vi "data-center-monitor.vi"() -> ()   [LabVIEW 2024]
doc: "Demonstrates how to implement advanced power measurement of harmonic parameters on a three-phase electrical power system, such as measurement of harmonic distortion factor, total harmonic distortion, harmonic power, etc. Measurement of harmonic parameters is based on a resampling algorithm."
uses:
  <vilib>/addons/Electrical Power/Power Measurement/subVIs/ep_Resampled Data.ctl
  <vilib>/Utility/error.llb/DialogType.ctl
  <vilib>/DAQmx/read.llb/DAQmx Read (Analog 1D Wfm NChan NSamp).vi
  <extravilib>/ChannelInstances/Tag-bool/Read.vi
  <extravilib>/ChannelInstances/Tag-bool/Write.vi
  <extravilib>/ChannelInstances/Tag-bool/Read With Abort.vi
  <extravilib>/ChannelInstances/Tag-bool/Write With Abort.vi
  <vilib>/DAQmx/create/channels.llb/DAQmx Create Channel (AI-Voltage-Basic).vi
  <vilib>/DAQmx/create/channels.llb/DAQmx Create Channel (AI-Current-Basic).vi
  <vilib>/DAQmx/configure/timing.llb/DAQmx Timing (Sample Clock).vi
  <extravilib>/ChannelInstances/Tag-bool/Instantiate.vi
  <vilib>/addons/Electrical Power/Basic/Measurement/Fundamental Vector (N Channels).vi
  <extravilib>/ChannelInstances/Tag-bool/EndpointRead.vi
  <extravilib>/ChannelInstances/Tag-bool/Endpoint.vi
  <vilib>/DAQmx/miscellaneous.llb/DAQmx Fill In Error Info.vi
  <resource>/objmgr/daqmx.rc
  <vilib>/addons/Electrical Power/Power Measurement/NI_EP_Power Measurement.lvlib
  <vilib>/addons/Electrical Power/Basic/NI_EP_Basic.lvlib
panel:
  in  "Display":T1(tab)
  in  "Configuration":enum32{"DAQmx", "Others"}(tab)
  in  "number of samples per channel":i32=10000
  in  "DAQmx sample rate [Hz]":dbl=50000.0 format="%0.2f"
  in  "current channels":tag="current-input/ai0:2"
  in  "maximum current value":dbl=0.002 format="%0.3f"
  in  "minimum current value":dbl=-0.002 format="%0.3f"
  in  "voltage channels":tag="voltage-input/ai0:2"
  in  "maximum voltage value":dbl=300.0 format="%0.2f"
  in  "minimum voltage value":dbl=-300.0 format="%0.2f"
  in  "frequency range [Hz]":cluster{"minimum":dbl, "maximum":dbl}={"minimum"=45.0, "maximum"=65.0}
  in  "samples per cycle":u16=192
  in  "cycles per block":u16=10
  in  "maximum harmonic  order":u16=50
  in  "distortion factor denominator":enum16{"Fundamental value", "Total value"}(ring)
  in  "filter for frequency measurement":T2={"enable filter? (T)"=TRUE, "passband edge frequency [Hz]"=65.0, "passband ripple [dB]"=0.1, "stopband edge frequency [Hz]"=85.0, "stopband attenuation [dB]"=60.0}
  out "Service Rack":cluster{dbl[], dbl[]}[](graph)
  out "PDU":cluster{dbl[], dbl[]}[](graph)
  out "V THD [%]":dbl[](array[numeric]) format="%#_2g"
  out "I THD [%]":dbl[](array[numeric]) format="%#_2g"
  out "Average Frequency [Hz]":dbl format="%#_3g"
  out "Power Usage":T3(graph)
  out "actual DAQmx \nsample rate  [Hz]":dbl
  out "average frequency [Hz]":dbl
  out "Waveforms":T4(graph)
  out "Voltage Harmonic Spectra":T5(graph)
  out "Current Harmonic Spectra":T5(graph)
  out "voltage total values":dbl[](array[numeric])
  out "voltage THD [%]":dbl[](array[numeric])
  out "voltage harmonic distortion factors [%]":dbl[][](array[numeric])
  out "current THD [%]":dbl[](array[numeric])
  out "total power value":T6
  out "harmonic power values":T7(array[cluster])
  out "power values":T3(array[cluster])
  out "Fundamental Voltage Vectors (Vrms)":cluster{dbl[], dbl[]}[](graph)
  out "Fundamental Current Vectors (Arms)":cluster{dbl[], dbl[]}[](graph)
  out "power history":T3(graph)
  in  "pause-update":bool
  in  "stop":bool
  # "Data Center Power Monitor Demo"
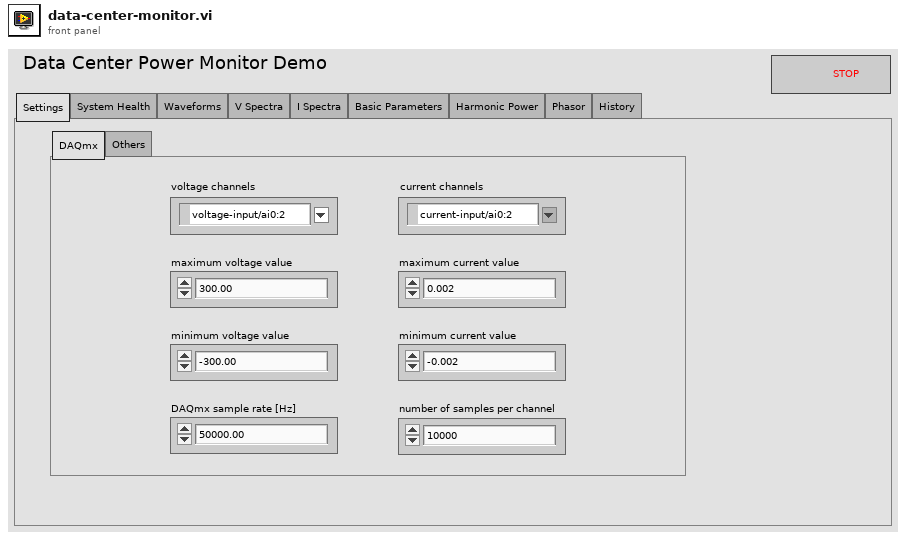
[diagram p1: front panel]
types:
  T1 = enum32{"Settings", "System Health", "Waveforms", "V Spectra", "I Spectra", "Basic Parameters", "Harmonic Power", "Phasor", "History"}
  T2 = cluster{"enable filter? (T)":bool, "passband edge frequency [Hz]":dbl, "passband ripple [dB]":dbl, "stopband edge frequency [Hz]":dbl, "stopband attenuation [dB]":dbl}
  T3 = cluster{"active power [W]":dbl, "apparent power [VA]":dbl, "reactive power [VAR]":dbl, "power factor":dbl}[]
  T4 = cluster{"positions [s]":dbl[], "resampled signal":dbl[]}[]
  T5 = cluster{"order 0":dbl, "delta order":dbl, "complex spectrum":dbl[]}[]
  T6 = cluster{"active power [W]":dbl, "apparent power [VA]":dbl, "reactive power [VAR]":dbl, "power factor":dbl}
  T7 = cluster{"active power [W]":dbl, "apparent power [VA]":dbl, "reactive power [VAR]":dbl, "power factor":dbl}[][]
  T8 = typedef "DialogType.ctl" = u16
  T9 = typedef "NI_EP_Power Measurement.lvlib/ep_Resampled Data.ctl" = cluster{"times [s]":dbl[], "resampled signal":dbl[]}
  T10 = cluster{"zero crossing times [s]":dbl[], "zero crossings per cycle":u8}
  T11 = typedef "Tag-bool.lvlib/))Channel.ctl" = refnum<queue>
  T12 = cluster{"order 0":dbl, "delta order":dbl, "complex spectrum":cdb[]}[]
  T13 = typedef "NI_EP_Basic.lvlib/basic_Power Value.ctl" = cluster{"active power [W]":dbl, "apparent power [VA]":dbl, "reactive power [VAR]":dbl, "power factor":dbl}
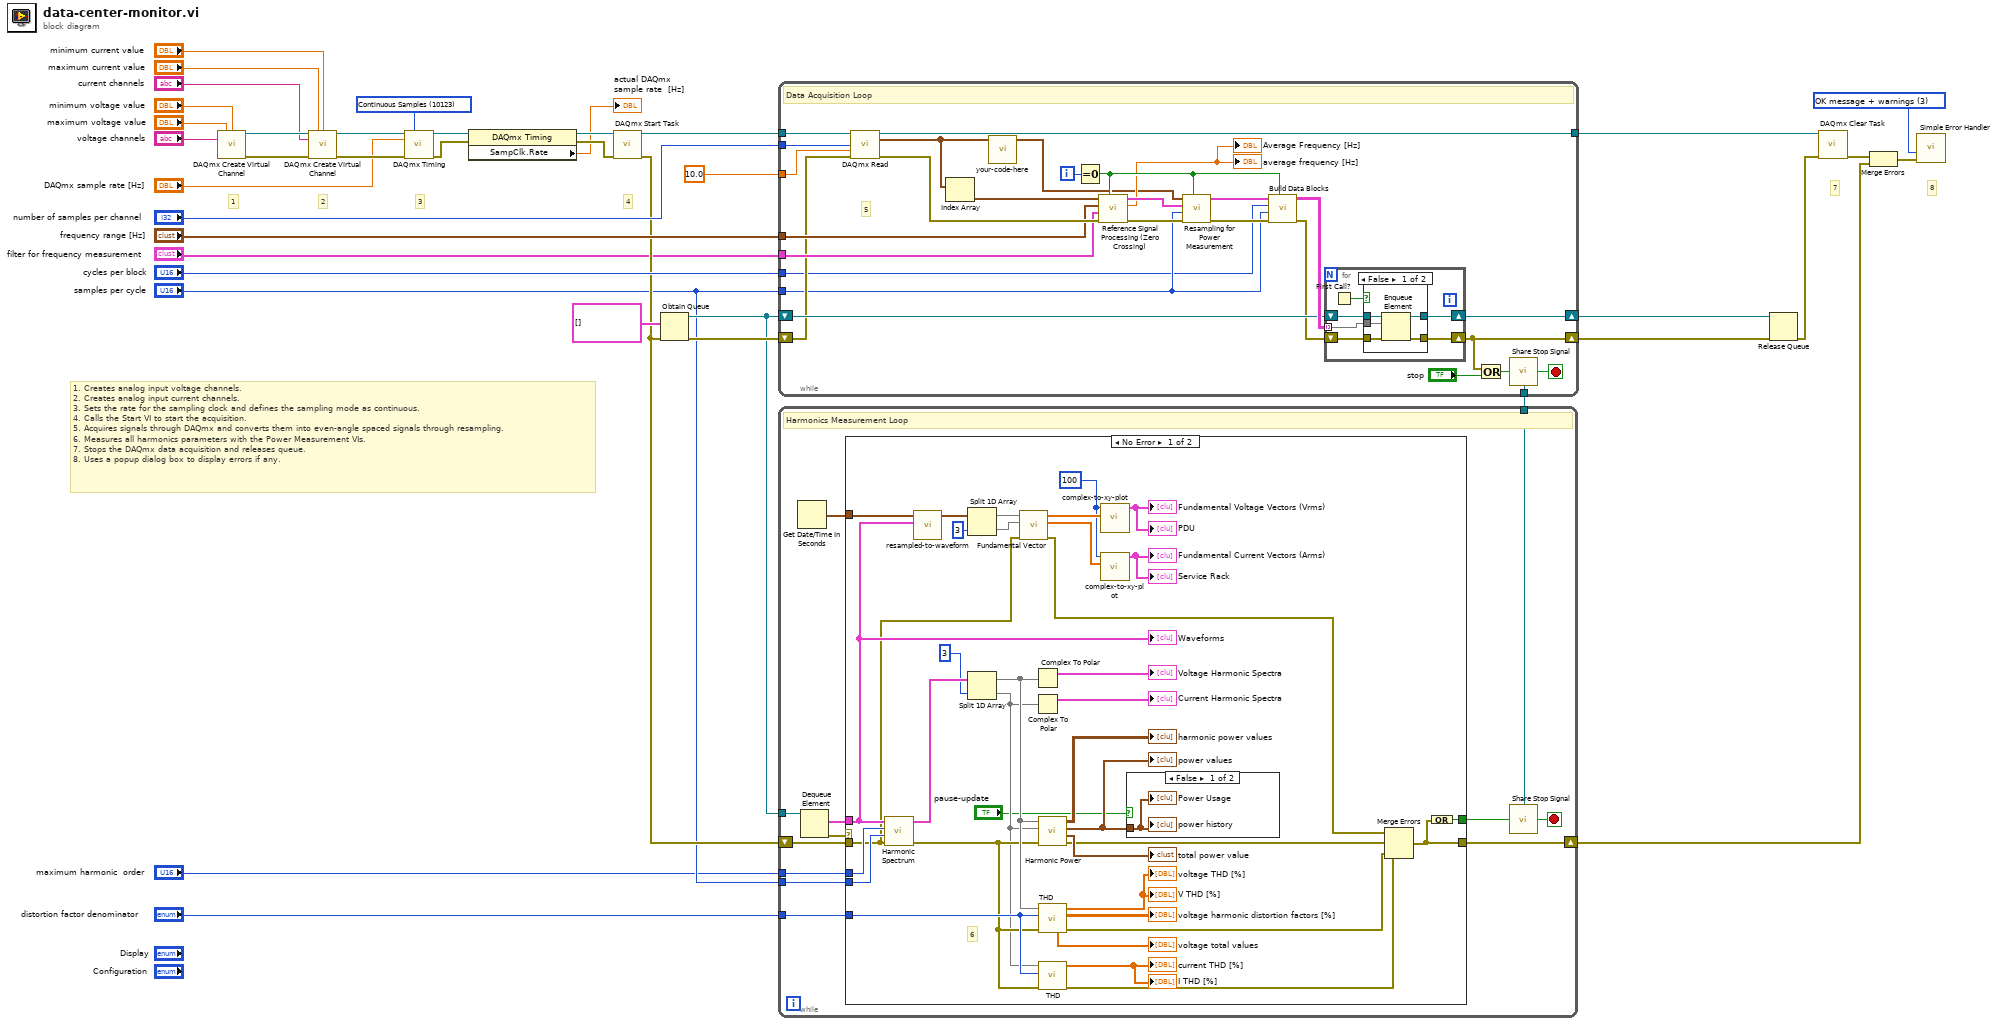
[diagram p0: block diagram]
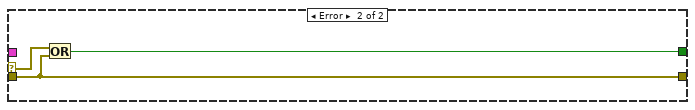
[diagram p3: hidden frame]
diagram:
  w6 = T8 3 items=["no dialog", "OK message", "continue or stop message", "OK message + warnings", "continue/stop + warnings"] ("type of dialog (OK msg:1)")
  w8 = 10123 items=["Finite Samples"=10178, "Continuous Samples"=10123, "Hardware Timed Single Point"=12522] ("sample mode")
  # "8"
  # "7"
  # "1. Creates analog input voltage channels.\n2. Creates analog input current channels.\n3. Sets the rate for the sampling clock and defines the sampling mode as continuous.\n4. Calls the Start VI to start the acquisition.\n5. Acquires signals through DAQmx and converts them into even-angle spaced signals through resampling. \n6. Measures all harmonics parameters with the Power Measurement VIs.\n7.\tStops the DAQmx data acquisition and releases queue.\n8. Uses a popup dialog box to display errors if any."
  # "4"
  # "3"
  # "2"
  # "1"
  n1 = call-poly <vilib>:"DAQmx Create Virtual Channel.vi"("maximum value"="maximum voltage value", "minimum value"="minimum voltage value", "physical channels"="voltage channels") -> ("task out"=w35:refnum<k21>, "error out"=w36:errorcluster)  [unwired: 11 in]
  n2 = call-poly <vilib>:"DAQmx Create Virtual Channel.vi"("task in"=w35, "maximum value"="maximum current value", "minimum value"="minimum current value", "physical channels"="current channels", "error in"=w36) -> ("task out"=w30:refnum<k21>, "error out"=w31:errorcluster)  [unwired: 9 in]
  n3 = call-poly <vilib>:"DAQmx Timing.vi"("task/channels in"=w30, "sample mode"=w8, "rate"="DAQmx sample rate [Hz]", "error in"=w31) -> ("task out"=w24:refnum<k21>, "error out"=w28:errorcluster)  [unwired: 10 in]
  n4 = property class="DAQmx Timing"(reference=w24, error in=w28) -> (reference out=w27:refnum<k21>, error out=w26:errorcluster, "SampClk.Rate"=→"actual DAQmx \nsample rate  [Hz]":dbl)
  n5 = call <vilib>:"DAQmx Start Task.vi"("task/channels in"=w27, "error in"=w26) -> ("task out"=w25:refnum<k21>, "error out"=w14:errorcluster)  [unwired: 12 in]
  n6 = Obtain Queue(element data type=T9[] [] ("resampled data"), error in (no error)=w14) -> (queue out=w15:refnum<queue>, error out=w19:errorcluster)  [unwired: 3 in, 1 out]
  n7 = while {
    tunnel: "number of samples per channel" -> [w67]
    tunnel: w25 -> [w68]
    tunnel: [w66] -> w21
    tunnel: "frequency range [Hz]" -> [w62]
    tunnel: "filter for frequency measurement" -> [w61]
    shift-right: [w52] -> w17
    shift-left: w15 -> [w54]
    shift-right: [w44] -> w4
    shift-left: w19 -> [w53]
    tunnel: "samples per cycle" -> [w51]
    tunnel: "cycles per block" -> [w50]
    tunnel: 10.0 ("timeout") -> [w46]
    tunnel: [w40] -> w1
    i -> [w64]
    stop <- w47 stop-if-true
    # "5"
    # "Data Acquisition Loop"
    n8 = call-poly <vilib>:"DAQmx Read.vi"("task/channels in"=w68, "number of samples per channel"=w67, "timeout"=w46, "error in"=w53) -> ("task out"=w66:refnum<k21>, "data"=w42:waveform(dbl)[], "error out"=w65:errorcluster)  [unwired: 9 in]
    n9 = Index Array(array=w42) -> (element=w63:waveform(dbl))  [unwired: 1 in]
    n10 = call "your-code-here.vi"("data in"=w42) -> ("data out"=w41:waveform(dbl)[])  [unwired: 10 in]
    n11 = Equal To 0?(x=w64) -> (x = 0?=w56:bool)
    n12 = call <vilib>:"Reference Signal Processing (Zero Crossing).vi"("reset? (F)"=w56, "error in (no error)"=w65, "filter for frequency measurement"=w61, "frequency range [Hz]"=w62, "reference signal"=w63) -> ("error out"=w60:errorcluster, "average frequency [Hz]"=→"average frequency [Hz]" →"Average Frequency [Hz]":dbl, "zero crossing information"=w59:T10)  [unwired: 3 in, 1 out]
    n13 = call <vilib>:"Resampling for Power Measurement.vi"("reset? (F)"=w56, "error in (no error)"=w60, "samples per cycle (192)"=w51, "trigger information"=w59, "data in"=w41) -> ("error out"=w58:errorcluster, "resampled data"=w57:T9[])  [unwired: 5 in]
    n14 = call <vilib>:"Build Data Blocks.vi"("reset? (F)"=w56, "error in (no error)"=w58, "samples per cycle (192)"=w51, "cycles per block (10)"=w50, "resampled data"=w57) -> ("error out"=w45:errorcluster, "data blocks"=w55:T9[][])  [unwired: 5 in]
    n15 = for {
      shift-right: [w72] -> w52
      shift-left: w54 -> [w73]
      shift-right: [w74] -> w44
      shift-left: w45 -> [w71]
      tunnel: w55 -> [w70] mode=indexing
      n16 = First Call?() -> (First Call?: T/F=w69:bool)
      n17 = case shown="False" w69 {
        tunnel: [w79 w80] -> w74
        tunnel: w73 -> [w78 w81]
        tunnel: [w77 w81] -> w72
        tunnel: w71 -> [w76 w80]
        tunnel: w70 -> [w75 _]
        frame False {
          n18 = Enqueue Element(queue=w78, element=w75, error in (no error)=w76) -> (queue out=w77:refnum<queue>, error out=w79:errorcluster)  [unwired: 1 in, 1 out]
        }
        frame True {
        }
      }
    }
    n19 = Or(x=w44, y="stop") -> (x .or. y?=w48:bool)
    n20 = call <vilib>:"Share Stop Signal.vi"("set stop (F)"=w48) -> ("channel"=w40:T11, "stop"=w47:bool)
  }
  n21 = while {
    shift-right: [w85] -> w10
    shift-left: w14 -> [w88]
    tunnel: w15 -> [w93]
    tunnel: "samples per cycle" -> [w91]
    tunnel: "maximum harmonic  order" -> [w90]
    tunnel: "distortion factor denominator" -> [w89]
    tunnel: w1 -> [w82]
    stop <- w86 stop-if-true
    # "Harmonics Measurement Loop"
    n22 = Get Date/Time In Seconds() -> (seconds since 1Jan1904=w83:timestamp)
    n23 = Dequeue Element(queue=w93) -> (element=w92:T9[], error out=w87:errorcluster)  [unwired: 2 in, 2 out]
    n24 = case shown="No Error" w87 {
      selector: w87 -> [_ w133]
      tunnel: w92 -> [w112 _]
      tunnel: w91 -> [w129 _]
      tunnel: w90 -> [w128 _]
      tunnel: w88 -> [w103 w132]
      tunnel: [w120 w132] -> w85
      tunnel: w89 -> [w125 _]
      tunnel: [w114 w131] -> w84
      tunnel: w83 -> [w111 _]
      frame No Error {
        w104 = 100
        # "6"
        n25 = call <vilib>:"Harmonic Spectrum.vi"("error in (no error)"=w103, "samples per cycle (192)"=w129, "maximum harmonic order (50)"=w128, "resampled data"=w112) -> ("error out"=w115:errorcluster, "harmonic spectra"=w127:T12)  [unwired: 6 in]
        n26 = call "resampled-to-waveform.vi"("resampled data"=w112, "current-timestamp"=w111) -> ("waveform data"=w109:waveform(dbl)[])  [unwired: 9 in]
        n27 = Split 1D Array(array=w109, index=3) -> (first subarray=w108:waveform(dbl)[], second subarray=w107:waveform(dbl)[])
        n28 = Split 1D Array(array=w127, index=3) -> (first subarray=w126:T12, second subarray=w100:T12)
        n29 = call-poly <vilib>:"Fundamental Vector.vi"("error in (no error)"=w103, "current waveforms"=w107, "voltage waveforms"=w108) -> ("error out"=w102:errorcluster, "current fundamental vectors"=w105:cdb[], "voltage fundamental vectors"=w106:cdb[])  [unwired: 5 in, 1 out]
        n30 = Complex To Polar(r * e^(i*theta)=w126) -> (r=→"Voltage Harmonic Spectra":T5)  [unwired: 1 out]
        n31 = Complex To Polar(r * e^(i*theta)=w100) -> (r=→"Current Harmonic Spectra":T5)  [unwired: 1 out]
        n32 = call <vilib>:"Harmonic Power.vi"("error in (no error)"=w115, "current spectra"=w100, "voltage spectra"=w126) -> ("error out"=w121:errorcluster, "total power value"=→"total power value":T13, "power values"=w101:T13[], "harmonic power values"=→"harmonic power values":T13[][])  [unwired: 5 in]
        "power values" <- w101
        n33 = call <vilib>:"THD.vi"("error in (no error)"=w115, "distortion factor denominator"=w125, "harmonic spectra"=w126) -> ("error out"=w116:errorcluster, "harmonic distortion factors [%]"=→"voltage harmonic distortion factors [%]":dbl[][], "THD [%]"=→"voltage THD [%]" →"V THD [%]":dbl[], "total values"=→"voltage total values":dbl[])  [unwired: 5 in]
        n34 = call <vilib>:"THD.vi"("error in (no error)"=w115, "distortion factor denominator"=w125, "harmonic spectra"=w100) -> ("error out"=w119:errorcluster, "THD [%]"=→"current THD [%]" →"I THD [%]":dbl[])  [unwired: 5 in, 2 out]
        n35 = call "complex-to-xy-plot.vi"("complex-vector"=w106, "number-of-points"=w104) -> ("xy-plot-output"=→"Fundamental Voltage Vectors (Vrms)" →"PDU":cluster{dbl[], dbl[]}[])  [unwired: 9 in]
        n36 = call "complex-to-xy-plot.vi"("complex-vector"=w105, "number-of-points"=w104) -> ("xy-plot-output"=→"Fundamental Current Vectors (Arms)" →"Service Rack":cluster{dbl[], dbl[]}[])  [unwired: 9 in]
        n37 = case shown="False" "pause-update" {
          tunnel: w101 -> [w130 _]
          frame False {
            "power history" <- w130
            "Power Usage" <- w130
          }
          frame True {
          }
        }
        n38 = Merge Errors(w102, w121, w116, w119) -> (w120:errorcluster)
        n39 = Compound Arithmetic op=OR(w120) -> (w114:bool)
        "Waveforms" <- w112
      }
      frame Error {
        n40 = Or(x=w133, y=w132) -> (x .or. y?=w131:bool)
      }
    }
    n41 = call <vilib>:"Share Stop Signal.vi"("set stop (F)"=w84, "channel"=w82) -> ("stop"=w86:bool)
  }
  n42 = Release Queue(queue=w17, error in (no error)=w4) -> (error out=w3:errorcluster)  [unwired: 1 in, 2 out]
  n43 = call <vilib>:"DAQmx Clear Task.vi"("task in"=w21, "error in"=w3) -> ("error out"=w2:errorcluster)  [unwired: 13 in]
  n44 = Merge Errors(w2, w10) -> (w9:errorcluster)
  n45 = call <vilib>:"Simple Error Handler.vi"("type of dialog (OK msg:1)"=w6, "error in (no error)"=w9) -> ()  [unwired: 3 in, 5 out]
